vi "BLtargetDealer.vi"(4 "n":string[](array[string]), 6 "TI":string[](array[string]), 9 "U":string[](array[string]), 10 "Z":string[](array[string]), 11 "Name":string[](array[string])) -> (2 "BLtargets":T1[](array[typedef]) {"n" min=0.02 max=0.5 step=0.01 format="%.2f"})   [LabVIEW 2022 SP3]
uses:
  BLTarget.ctl
  119a32a6-1c17-bf47-9c76-87b11b2d3316.vi
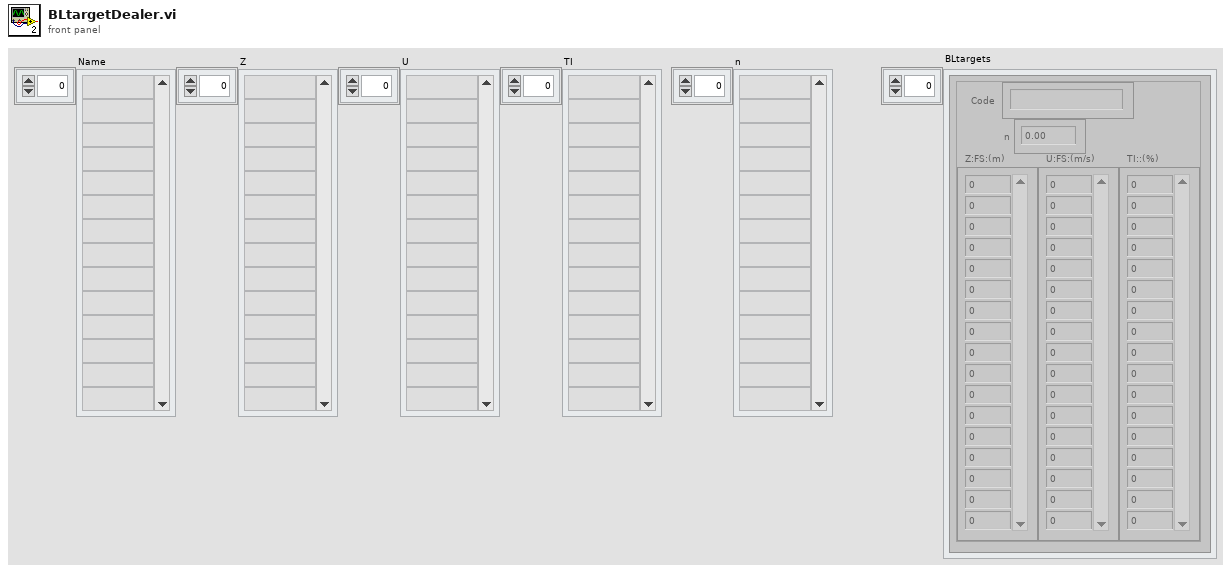
[diagram p1: front panel]
types:
  T1 = typedef "BLTarget.ctl" = cluster{"Code":string, "n":dbl, "Z:FS:(m)":dbl[], "U:FS:(m/s)":dbl[], "TI::(%)":dbl[]}
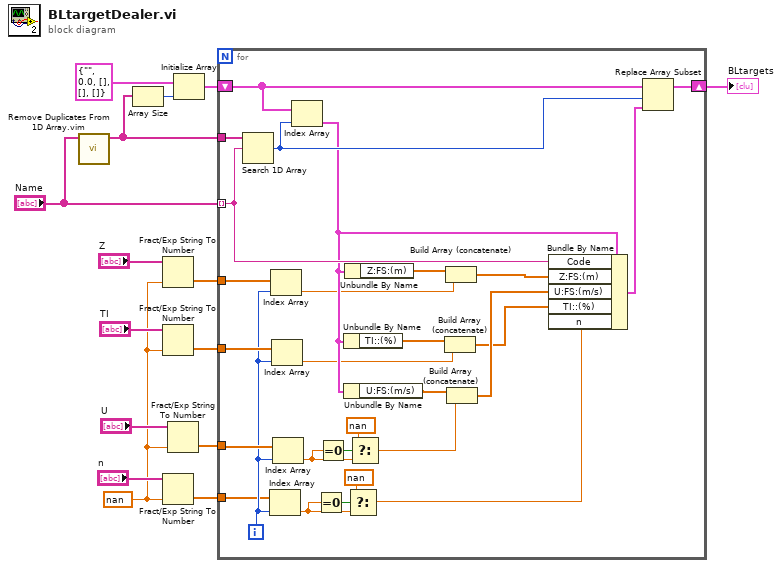
[diagram p0: block diagram]
diagram:
  w1 = nan ("default (0 DBL)")
  n1 = call "Remove Duplicates From 1D Array.vim"("array"="Name") -> ("array with duplicates removed"=w10:string[])  [unwired: 10 in]
  n2 = Array Size(array=w10) -> (size(s)=w9:i32)
  n3 = Fract/Exp String To Number(string="Z", default (0 dbl)=w1) -> (number=w6:dbl[])  [unwired: 2 in, 1 out]
  n4 = Fract/Exp String To Number(string="TI", default (0 dbl)=w1) -> (number=w4:dbl[])  [unwired: 2 in, 1 out]
  n5 = Fract/Exp String To Number(string="n", default (0 dbl)=w1) -> (number=w2:dbl[])  [unwired: 2 in, 1 out]
  n6 = Fract/Exp String To Number(string="U", default (0 dbl)=w1) -> (number=w5:dbl[])  [unwired: 2 in, 1 out]
  n7 = Initialize Array(T1 {"Code"="", "n"=0.0, "Z:FS:(m)"=[], "U:FS:(m/s)"=[], "TI::(%)"=[]} ("Cluster"), w9) -> (w8:T1[])
  n8 = for {
    tunnel: "Name" -> [w36] mode=indexing
    tunnel: w10 -> [w43]
    shift-right: [w41] -> w7
    shift-left: w8 -> [w42]
    tunnel: w6 -> [w30]
    tunnel: w5 -> [w29]
    tunnel: w4 -> [w28]
    tunnel: w2 -> [w24]
    i -> [w27]
    n9 = Search 1D Array(1D array=w43, element=w36) -> (index of element=w40:i32)  [unwired: 1 in]
    n10 = Index Array(array=w24, index=w27) -> (element=w21:dbl)
    n11 = Index Array(array=w30, index=w27) -> (element=w26:dbl)
    n12 = Index Array(array=w28, index=w27) -> (element=w25:dbl)
    n13 = Index Array(array=w29, index=w27) -> (element=w17:dbl)
    n14 = Index Array(array=w42, index=w40) -> (element=w35:T1)
    n15 = Equal To 0?(x=w21) -> (x = 0?=w22:bool)
    n16 = Equal To 0?(x=w17) -> (x = 0?=w20:bool)
    n17 = Unbundle By Name(w35) -> ("TI::(%)"=w33:dbl[])
    n18 = Unbundle By Name(w35) -> ("U:FS:(m/s)"=w34:dbl[])
    n19 = Unbundle By Name(w35) -> ("Z:FS:(m)"=w38:dbl[])
    n20 = Select(t=nan, s=w22, f=w21) -> (s? t:f=w23:dbl)
    n21 = Select(t=nan, s=w20, f=w17) -> (s? t:f=w16:dbl)
    n22 = Build Array (concatenate)(w33, w25) -> (w31:dbl[])
    n23 = Build Array (concatenate)(w38, w26) -> (w37:dbl[])
    n24 = Build Array (concatenate)(w34, w16) -> (w32:dbl[])
    n25 = Bundle By Name(cluster=w35, "Code"=w36, "Z:FS:(m)"=w37, "U:FS:(m/s)"=w32, "TI::(%)"=w31, "n"=w23) -> (w39:T1)
    n26 = Replace Array Subset(array=w42, new element=w39, index=w40) -> (w41:T1[])
  }
  "BLtargets" <- w7
